vi "Init SMC100.vi"(8 "error in (no error)":errorcluster caption="entrée d'erreur (pas d'erreur)", 11 "UI SA en entrée":refnum<class "UI SmarAct.lvclass">) -> (0 "error out":errorcluster caption="sortie d'erreur", 1 "StageIdentifier":string, 2 "ControllerVersion":string, 3 "UI SA en sortie":refnum<class "UI SmarAct.lvclass">, 5 "Erreur":bool)   [LabVIEW 2024, in "UI SmarAct.lvclass"]
uses:
  UI SmarAct.lvclass
  C:/Program Files (x86)/National Instruments/LabVIEW 2024/vi.lib/addons/_Workers/Library/Classes/Worker/Worker.lvclass
  UI SmarAct.lvclass/UI SmarAct.ctl
  Status Platine Newport/rqp_Start Status.ctl
  Status Platine Newport/rqp_Stop Status.ctl
  <vilib>/Utility/error.llb/Error Cluster From Error Code.vi
  Newport.SMC100.CommandInterface
  <vilib>/ErrorRing/Error Ring.xnode
  Status Platine Newport/Status Platine Newport.lvclass
panel:
  out "errstring 2":string
  out "errstring":string
  out "Error":i32
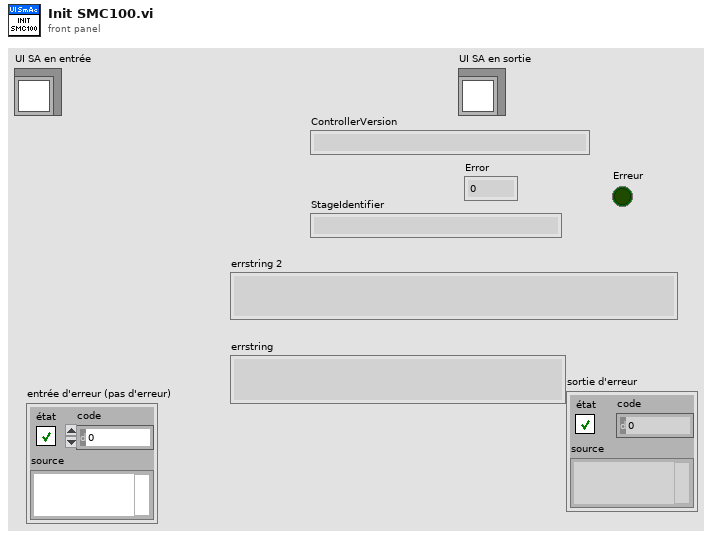
[diagram p1: front panel]
types:
  T1 = typedef "Status Platine Newport.lvclass/rqp_Start Status.ctl" = cluster{"Adresse SMC100":i32, "SMC100 Reference":refnum<k24>, "RefnumStatus Platine":refnum<vi>}
  T2 = enum8{"Enabled", "Disabled", "Disabled and Grayed Out"}
  T3 = typedef "Status Platine Newport.lvclass/rqp_Stop Status.ctl" = cluster{"RefnumStatus Platine":refnum<vi>}
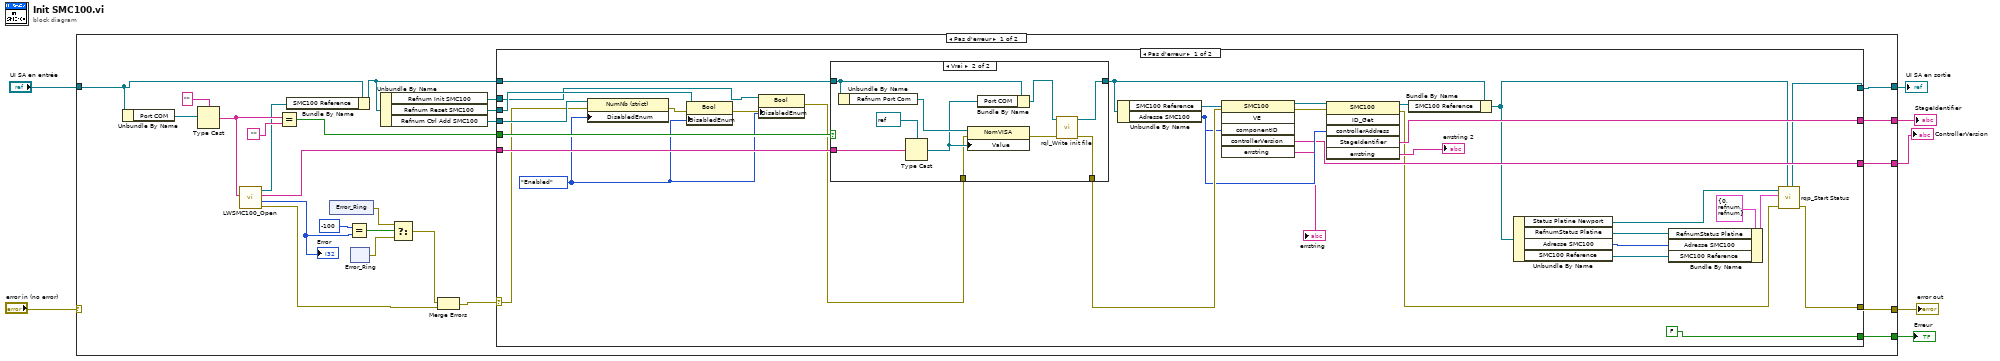
[diagram p0: block diagram]
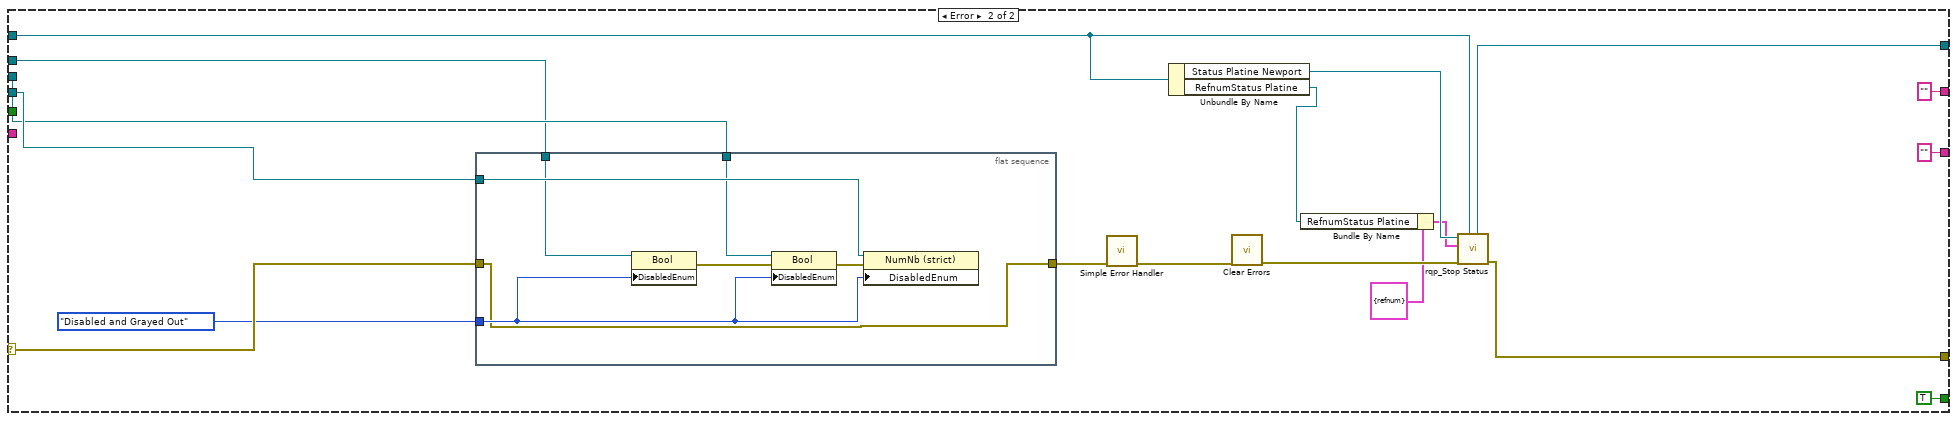
[diagram p3: hidden frame]
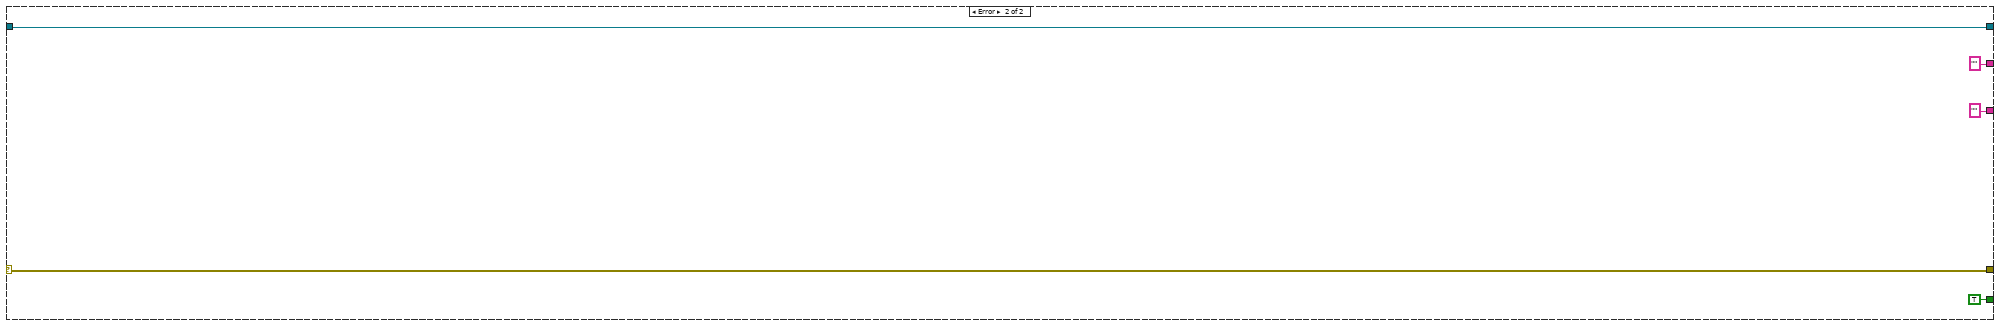
[diagram p4: hidden frame]
diagram:
  n1 = case shown="Pas d'erreur" "error in (no error)" {
    selector: "error in (no error)" -> [_ w113]
    tunnel: [w26 w113] -> w6
    tunnel: [w25 w112] -> w4
    tunnel: "UI SA en entrée" -> [w16 w112]
    tunnel: [w12 "" ("controllerVersion")] -> w3
    tunnel: [w11 "" ("StageIdentifier")] -> w2
    tunnel: [w10 TRUE] -> w1
    frame No Error {
      n2 = Unbundle By Name(w16) -> ("Port COM"=w32:refnum<visa-resource-name>)
      n3 = Type Cast(type="", x=w32) -> (*(type *) &x=w30:string)
      n4 = call "LWSMC100_Open.vi"("Instrument Key IN"=w30) -> ("error out"=w22:errorcluster, "Error"=w24:i32, "Instrument Key OUT"=w28:string, "CommandInterfaceSMC100.SMC100"=w13:refnum<k24>)  [unwired: 3 in]
      "Error" <- w24
      n5 = Equal?(x=w30, y="") -> (x = y?=w27:bool)
      n6 = Bundle By Name(cluster=w16, "SMC100 Reference"=w13) -> (w14:refnum<class "UI SmarAct.lvclass">)
      n7 = xnode ("Error_Ring")() -> ("sortie d'erreur"=w18:errorcluster)
      n8 = Equal?(x=-100, y=w24) -> (x = y?=w20:bool)
      n9 = xnode ("Error_Ring")() -> ("sortie d'erreur"=w19:errorcluster)
      n10 = Unbundle By Name(w14) -> ("Refnum Init SMC100"=w8:refnum<vi>, "Refnum Reset SMC100"=w9:refnum<vi>, "Refnum Ctrl Add SMC100"=w15:refnum<vi>)
      n11 = Select(t=w18, s=w20, f=w19) -> (s? t:f=w17:errorcluster)
      n12 = Merge Errors(w17, w22) -> (w21:errorcluster)
      n13 = case shown="Pas d'erreur" w21 {
        selector: w21 -> [w67 w95]
        tunnel: w28 -> [w71 _]
        tunnel: w27 -> [w70 _]
        tunnel: w14 -> [w69 w96]
        tunnel: [w52 w92] -> w26
        tunnel: [w49 w91] -> w25
        tunnel: w15 -> [w68 w98]
        tunnel: [w59 "" ("controllerVersion")] -> w12
        tunnel: [w58 "" ("StageIdentifier")] -> w11
        tunnel: [FALSE TRUE] -> w10
        tunnel: w9 -> [w44 w85]
        tunnel: w8 -> [w43 w84]
        frame No Error {
          w40 = T2."Enabled" ("Désactivée")
          n14 = property class="NumNb (strict)"(reference=w68, error in=w67, "DisabledEnum"=w40) -> (error out=w42:errorcluster)  [unwired: 1 out]
          n15 = property class="Bool"(reference=w44, error in=w42, "DisabledEnum"=w40) -> (error out=w41:errorcluster)  [unwired: 1 out]
          n16 = property class="Bool"(reference=w43, error in=w41, "DisabledEnum"=w40) -> (error out=w45:errorcluster)  [unwired: 1 out]
          n17 = case shown="Vrai" w70 {
            tunnel: w71 -> [_ w82]
            tunnel: w69 -> [w73 w81]
            tunnel: [w73 w76] -> w66
            tunnel: w45 -> [w72 w78]
            tunnel: [w72 w74] -> w63
            frame False {
            }
            frame True {
              n18 = Unbundle By Name(w81) -> ("Refnum Port Com"=w80:refnum<vi>)
              n19 = Type Cast(type=refnum<visa-resource-name> refnum ("Response Cases.Port COM"), x=w82) -> (*(type *) &x=w79:refnum<visa-resource-name>)
              n20 = property class="NomVISA"(reference=w80, error in=w78, "Value"=w79) -> (error out=w75:errorcluster)  [unwired: 1 out]
              n21 = Bundle By Name(cluster=w81, "Port COM"=w79) -> (w77:refnum<class "UI SmarAct.lvclass">)
              n22 = call "rql_Write init file.vi"("error in"=w75, "UI SmarAct in"=w77) -> ("error out"=w74:errorcluster, "dup UI SmarAct out"=w76:refnum<class "UI SmarAct.lvclass">)  [unwired: 8 in]
            }
          }
          n23 = Unbundle By Name(w66) -> ("SMC100 Reference"=w65:refnum<k24>, "Adresse SMC100"=w60:i32)
          n24 = invoke class="SMC100" method="VE"(reference=w65, error in=w63, "componentID"=w60) -> (reference out=w64:refnum<k24>, error out=w62:errorcluster, "controllerVersion"=w59:string, "errstring"=→"errstring":string)  [unwired: 3 in, 2 out]
          n25 = invoke class="SMC100" method="ID_Get"(reference=w64, error in=w62, "controllerAddress"=w60) -> (reference out=w61:refnum<k24>, error out=w53:errorcluster, "StageIdentifier"=w58:string, "errstring"=→"errstring 2":string)  [unwired: 3 in, 2 out]
          n26 = Bundle By Name(cluster=w66, "SMC100 Reference"=w61) -> (w50:refnum<class "UI SmarAct.lvclass">)
          n27 = Unbundle By Name(w50) -> ("Status Platine Newport"=w51:refnum<class "Status Platine Newport.lvclass">, "RefnumStatus Platine"=w39:refnum<vi>, "Adresse SMC100"=w47:i32, "SMC100 Reference"=w46:refnum<k24>)
          n28 = Bundle By Name(cluster=T1 {"Adresse SMC100"=0, "SMC100 Reference"=refnum, "RefnumStatus Platine"=refnum} ("Data in"), "RefnumStatus Platine"=w39, "Adresse SMC100"=w47, "SMC100 Reference"=w46) -> (w48:T1)
          n29 = call "rqp_Start Status.vi"("Caller in"=w50, "error in"=w53, "Data in"=w48, "Status Platine Newport in"=w51) -> ("error out"=w52:errorcluster, "dup Caller out"=w49:refnum<class "UI SmarAct.lvclass">)  [unwired: 5 in, 1 out]
        }
        frame Error {
          n30 = flat-sequence {
            tunnel: w98 -> [w108]
            tunnel: w95 -> [w102]
            tunnel: [w102] -> w94
            tunnel: T2."Disabled and Grayed Out" ("Désactivée") -> [w105]
            tunnel: w85 -> [w104]
            tunnel: w84 -> [w103]
            frame #0 {
              n31 = property class="Bool"(reference=w103, "DisabledEnum"=w105) -> (error out=w107:errorcluster)  [unwired: 1 in, 1 out]
              n32 = property class="Bool"(reference=w104, error in=w107, "DisabledEnum"=w105) -> (error out=w106:errorcluster)  [unwired: 1 out]
              n33 = property class="NumNb (strict)"(reference=w108, error in=w106, "DisabledEnum"=w105) -> ()  [unwired: 2 out]
            }
          }
          n34 = call <vilib>:"Simple Error Handler.vi"("error in (no error)"=w94) -> ("error out"=w101:errorcluster)  [unwired: 4 in, 4 out]
          n35 = Unbundle By Name(w96) -> ("Status Platine Newport"=w90:refnum<class "Status Platine Newport.lvclass">, "RefnumStatus Platine"=w87:refnum<vi>)
          n36 = call <vilib>:"Clear Errors.vi"("error in (no error)"=w101) -> ("error out"=w93:errorcluster)  [unwired: 5 in, 1 out]
          n37 = Bundle By Name(cluster=T3 {"RefnumStatus Platine"=refnum} ("Data in"), "RefnumStatus Platine"=w87) -> (w88:T3)
          n38 = call "rqp_Stop Status.vi"("Caller in"=w96, "error in"=w93, "Data in"=w88, "Status Platine Newport in"=w90) -> ("error out"=w92:errorcluster, "dup Caller out"=w91:refnum<class "UI SmarAct.lvclass">)  [unwired: 5 in, 1 out]
        }
      }
    }
    frame Error {
    }
  }
  "error out" <- w6
  "UI SA en sortie" <- w4
  "ControllerVersion" <- w3
  "StageIdentifier" <- w2
  "Erreur" <- w1
